vi "Edit Assert Settings.vi"   [LabVIEW 2018, in "Assert API Components.lvlib"]
uses:
  Assert API Components/Assert API Components.lvlib
  <vilib>/Utility/sysdir.llb/System Directory Type.ctl
types:
  T1 = typedef "System Directory Type.ctl" = i32
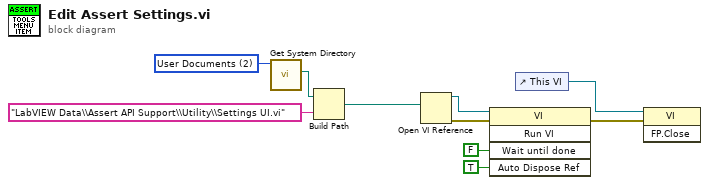
[diagram p0: block diagram]
diagram:
  w10 = T1 2 items=["User Home"=0, "User Desktop"=1, "User Documents"=2, "User Application Data"=3, "User Preferences"=4, "User Temporary"=5, "Public Documents"=6, "Public Application Data"=7, "Public Preferences"=8, "Public Cache"=13, "System Core Libraries"=9, "System Installed Libraries"=10, "Application Files"=11, "Boot Volume Root"=12] ("system directory type")
  n1 = call <vilib>:"Get System Directory.vi"("system directory type"=w10) -> ("system directory"=w9:path)  [unwired: 10 in]
  n2 = Build Path(base path=w9, name or relative path="LabVIEW Data\\Assert API Support\\Utility\\Settings UI.vi") -> (appended path=w7:path)
  n3 = Open VI Reference(vi path=w7) -> (vi reference=w6:refnum<vi>, error out=w5:errorcluster)  [unwired: 5 in]
  n4 = invoke class="VI" method="Run VI"(reference=w6, error in=w5, "Wait until done"=FALSE ("Wait Until Done"), "Auto Dispose Ref"=TRUE ("Auto Dispose Reference")) -> (error out=w2:errorcluster)  [unwired: 1 in, 4 out]
  n5 = control-ref of="This VI"() -> (w1:refnum<vi>)
  n6 = invoke class="VI" method="FP.Close"(reference=w1, error in=w2) -> ()  [unwired: 1 in, 3 out]
